vi "auto_rampnav.vi"(11 "Distance":dbl=7000.0) -> (3 "Complete":bool)   [LabVIEW 2010, in "LASA Beta.lvrbt"]
uses:
  LASA Beta.lvrbt
  op-run.vi
  op-read.vi
  <vilib>/NXT/Dual Mode Library/Display/drawNumber.vi
  <vilib>/NXT/Dual Mode Library/Display/drawText_center.vi
  <vilib>/NXT/Dual Mode Library/Waits/Wait_Num(msec).vi
panel:
  in  "Speed":dbl=40.0
  # "Measured in encoder counts, from wall start to 4th box"
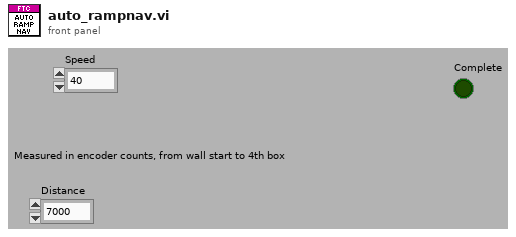
[diagram p1: front panel]
types:
  T1 = enum16{"Move Forward", "Move Left", "Allign To Ramp", "Orient To Ramp", "Climb Ramp", "Exit"}
  T2 = typedef "LVHSConnector.ctl" = cluster{"Hardware":string, "Flattened String":string}
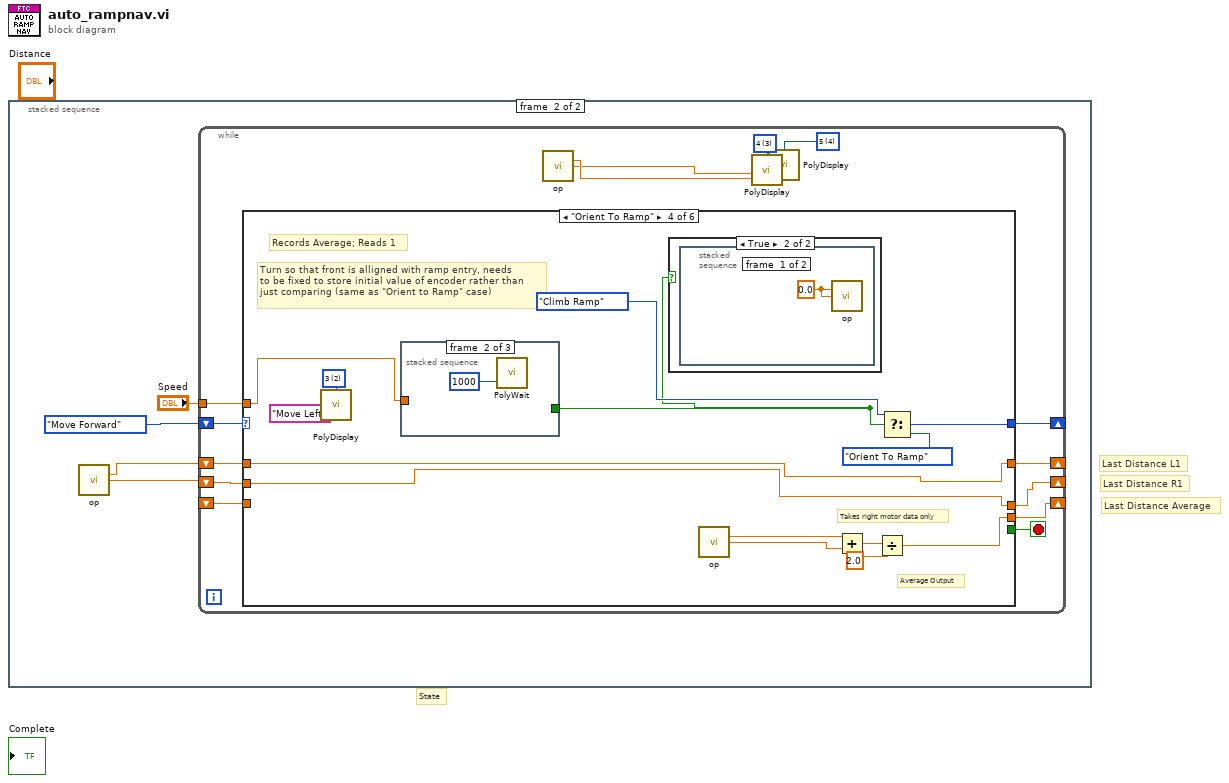
[diagram p0: block diagram]
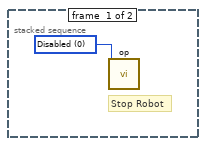
[diagram p2: hidden frame]
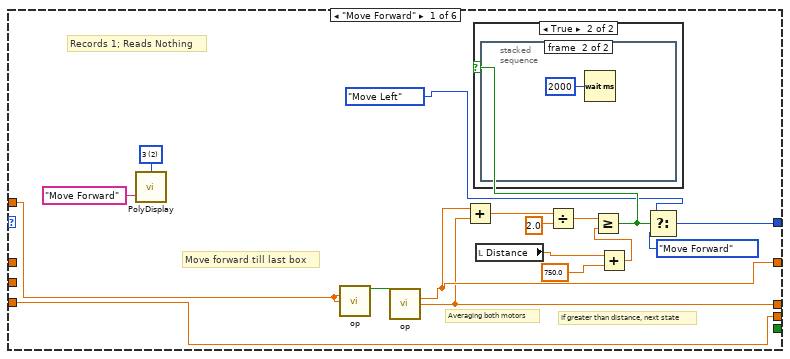
[diagram p3: hidden frame]
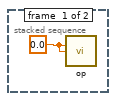
[diagram p5: hidden frame]
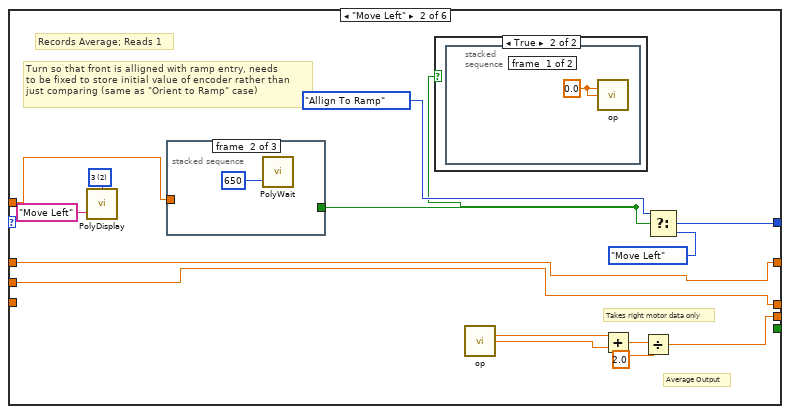
[diagram p6: hidden frame]
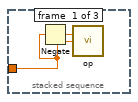
[diagram p7: hidden frame]
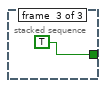
[diagram p8: hidden frame]
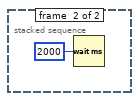
[diagram p10: hidden frame]
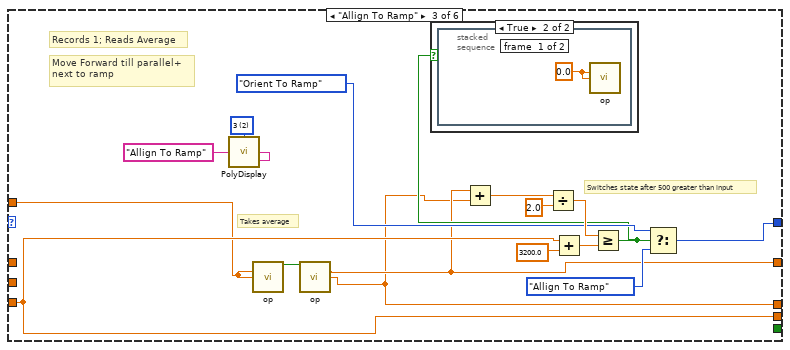
[diagram p11: hidden frame]
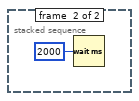
[diagram p13: hidden frame]
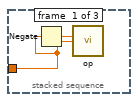
[diagram p14: hidden frame]
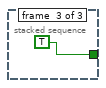
[diagram p15: hidden frame]
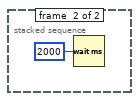
[diagram p17: hidden frame]
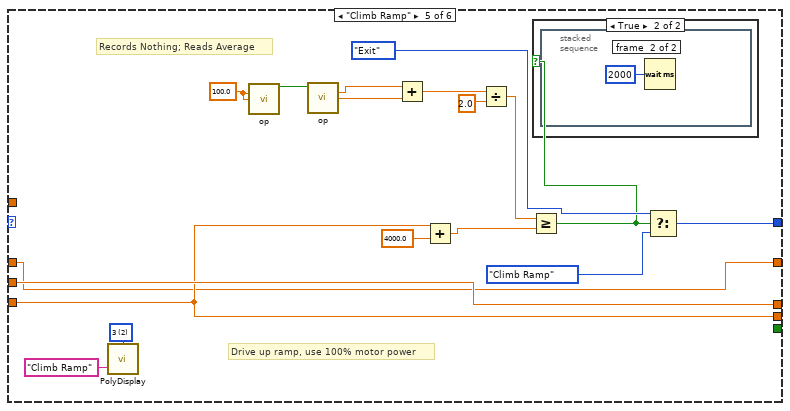
[diagram p18: hidden frame]
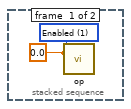
[diagram p20: hidden frame]
diagram:
  # "Last Distance Average"
  # "Last Distance R1"
  # "Last Distance L1"
  # "State"
  n1 = stacked-sequence {
    frame #0 {
      w1 = u16 0 items=["Disabled", "Enabled", "Initialize", "Read Only"] ("Status")
      # "Stop Robot"
      n2 = call-poly "op.vi"("Left Drive"=w1) -> ()  [unwired: 14 in, 1 out]
    }
    frame #1 {
      n3 = call-poly "op.vi"() -> ("Encoder Left Drive"=w4:dbl, "Encoder Right Drive"=w3:dbl)  [unwired: 9 in, 5 out]
      n4 = while {
        shift-right: [w19] -> _
        shift-left: T1."Move Forward" -> [w20]
        shift-right: [w8] -> _
        shift-left: w4 -> [w17]
        shift-right: [w12] -> _
        shift-left: w3 -> [w16]
        shift-right: [w11] -> _
        shift-left: _ -> [w15]
        tunnel: "Speed" -> [w6]
        stop <- w18 stop-if-true
        w13 = i16 4 items=["1", "2", "3", "4", "5", "6", "7", "8"] ("Line")
        w14 = i16 3 items=["1", "2", "3", "4", "5", "6", "7", "8"] ("Line")
        n5 = case shown="\"Orient To Ramp\"" w20 {
          tunnel: [w34 w52 w71 w90 w110 T1."Exit"] -> w19
          tunnel: [_ _ _ _ _ w125] -> w18
          tunnel: w17 -> [_ w42 _ w80 w98 w120]
          tunnel: [w23 w48 w61 w86 w107 w124] -> w12
          tunnel: [w32 w50 w68 w88 w106 w123] -> w11
          tunnel: w16 -> [_ w48 _ w86 w107 w124]
          tunnel: w15 -> [w32 _ w68 _ w106 w123]
          tunnel: [w24 w42 w62 w80 w98 w120] -> w8
          tunnel: w6 -> [w21 w40 w60 w78 _ _]
          frame "Move Forward" {
            w31 = i16 2 items=["1", "2", "3", "4", "5", "6", "7", "8"] ("Line")
            # "If greater than distance, next state"
            # "Averaging both motors"
            # "Records 1; Reads Nothing"
            # "Move forward till last box"
            n6 = call-poly <vilib>:"PolyDisplay.vi"("Text"="Move Forward", "Line"=w31) -> ()  [unwired: 2 in, 1 out]
            n7 = call-poly "op.vi"("Left Drive"=w21, "Right Drive"=w21) -> ("Chain OUT"=w22:bool)  [unwired: 13 in]
            n8 = call-poly "op.vi"("Chain IN"=w22) -> ("Encoder Left Drive"=w24:dbl, "Encoder Right Drive"=w23:dbl)  [unwired: 8 in, 5 out]
            n9 = Add(x=w24, y=w23) -> (x+y=w37:dbl)
            n10 = local read "Distance"() -> (w27:dbl)
            n11 = Divide(x=w37, y=2.0) -> (x/y=w33:dbl)
            n12 = Add(x=w27, y=750.0) -> (x+y=w25:dbl)
            n13 = Greater Or Equal?(x=w33, y=w25) -> (x >= y?=w29:bool)
            n14 = case shown="True" w29 {
              frame False {
              }
              frame True {
                n15 = stacked-sequence {
                  frame #0 {
                    w38 = 0.0 ("y")
                    n16 = call-poly "op.vi"("Left Drive"=w38, "Right Drive"=w38) -> ()  [unwired: 13 in, 1 out]
                  }
                  frame #1 {
                    n17 = Wait (ms)(milliseconds to wait=u32 2000) -> ()  [unwired: 1 out]
                  }
                }
              }
            }
            n18 = Select(t=T1."Move Left", s=w29, f=T1."Move Forward") -> (s? t:f=w34:T1)
          }
          frame "Move Left" {
            w47 = i16 2 items=["1", "2", "3", "4", "5", "6", "7", "8"] ("Line")
            # "Takes right motor data only"
            # "Average Output"
            # "Records Average; Reads 1"
            # "Turn so that front is alligned with ramp entry, needs\nto be fixed to store initial value of encoder rather than \njust comparing (same as \"Orient to Ramp\" case)"
            n19 = call-poly <vilib>:"PolyDisplay.vi"("Text"="Move Left", "Line"=w47) -> ()  [unwired: 2 in, 1 out]
            n20 = stacked-sequence {
              tunnel: [_ _ TRUE] -> w41
              tunnel: w40 -> [w55 _ _]
              frame #0 {
                n21 = Negate(x=w55) -> (-x=w54:dbl)
                n22 = call-poly "op.vi"("Left Drive"=w54, "Right Drive"=w55) -> ()  [unwired: 13 in, 1 out]
              }
              frame #1 {
                n23 = call-poly <vilib>:"PolyWait.vi"("Time (100 msec)"=u32 650) -> ()  [unwired: 3 in, 1 out]
              }
              frame #2 {
              }
            }
            n24 = case shown="True" w41 {
              frame False {
              }
              frame True {
                n25 = stacked-sequence {
                  frame #0 {
                    w58 = 0.0 ("y")
                    n26 = call-poly "op.vi"("Left Drive"=w58, "Right Drive"=w58) -> ()  [unwired: 13 in, 1 out]
                  }
                  frame #1 {
                    n27 = Wait (ms)(milliseconds to wait=u32 2000) -> ()  [unwired: 1 out]
                  }
                }
              }
            }
            n28 = call-poly "op.vi"() -> ("Encoder Left Drive"=w44:dbl, "Encoder Right Drive"=w43:dbl)  [unwired: 9 in, 5 out]
            n29 = Add(x=w44, y=w43) -> (x+y=w51:dbl)
            n30 = Divide(x=w51, y=2.0) -> (x/y=w50:dbl)
            n31 = Select(t=T1."Allign To Ramp", s=w41, f=T1."Move Left") -> (s? t:f=w52:T1)
          }
          frame "Allign To Ramp" {
            w67 = i16 2 items=["1", "2", "3", "4", "5", "6", "7", "8"] ("Line")
            # "Switches state after 500 greater than input"
            # "Takes average"
            # "Records 1; Reads Average"
            # "Move Forward till parallel+\nnext to ramp"
            n32 = call-poly <vilib>:"PolyDisplay.vi"("Text"="Allign To Ramp", "Line"=w67) -> ()  [unwired: 2 in, 1 out]
            n33 = call-poly "op.vi"("Left Drive"=w60, "Right Drive"=w60) -> ("Chain OUT"=w63:bool)  [unwired: 13 in]
            n34 = call-poly "op.vi"("Chain IN"=w63) -> ("Encoder Left Drive"=w62:dbl, "Encoder Right Drive"=w61:dbl)  [unwired: 8 in, 5 out]
            n35 = Add(x=w62, y=w61) -> (x+y=w75:dbl)
            n36 = Divide(x=w75, y=2.0) -> (x/y=w73:dbl)
            n37 = Add(x=w68, y=3200.0) -> (x+y=w70:dbl)
            n38 = Greater Or Equal?(x=w73, y=w70) -> (x >= y?=w64:bool)
            n39 = case shown="True" w64 {
              frame False {
              }
              frame True {
                n40 = stacked-sequence {
                  frame #0 {
                    w76 = 0.0 ("y")
                    n41 = call-poly "op.vi"("Left Drive"=w76, "Right Drive"=w76) -> ()  [unwired: 13 in, 1 out]
                  }
                  frame #1 {
                    n42 = Wait (ms)(milliseconds to wait=u32 2000) -> ()  [unwired: 1 out]
                  }
                }
              }
            }
            n43 = Select(t=T1."Orient To Ramp", s=w64, f=T1."Allign To Ramp") -> (s? t:f=w71:T1)
          }
          frame "Orient To Ramp" {
            w85 = i16 2 items=["1", "2", "3", "4", "5", "6", "7", "8"] ("Line")
            # "Takes right motor data only"
            # "Average Output"
            # "Records Average; Reads 1"
            # "Turn so that front is alligned with ramp entry, needs\nto be fixed to store initial value of encoder rather than \njust comparing (same as \"Orient to Ramp\" case)"
            n44 = call-poly <vilib>:"PolyDisplay.vi"("Text"="Move Left", "Line"=w85) -> ()  [unwired: 2 in, 1 out]
            n45 = stacked-sequence {
              tunnel: [_ _ TRUE] -> w79
              tunnel: w78 -> [w93 _ _]
              frame #0 {
                n46 = Negate(x=w93) -> (-x=w92:dbl)
                n47 = call-poly "op.vi"("Left Drive"=w92, "Right Drive"=w93) -> ()  [unwired: 13 in, 1 out]
              }
              frame #1 {
                n48 = call-poly <vilib>:"PolyWait.vi"("Time (100 msec)"=u32 1000) -> ()  [unwired: 3 in, 1 out]
              }
              frame #2 {
              }
            }
            n49 = case shown="True" w79 {
              frame False {
              }
              frame True {
                n50 = stacked-sequence {
                  frame #0 {
                    w96 = 0.0 ("y")
                    n51 = call-poly "op.vi"("Left Drive"=w96, "Right Drive"=w96) -> ()  [unwired: 13 in, 1 out]
                  }
                  frame #1 {
                    n52 = Wait (ms)(milliseconds to wait=u32 2000) -> ()  [unwired: 1 out]
                  }
                }
              }
            }
            n53 = call-poly "op.vi"() -> ("Encoder Left Drive"=w82:dbl, "Encoder Right Drive"=w81:dbl)  [unwired: 9 in, 5 out]
            n54 = Add(x=w82, y=w81) -> (x+y=w89:dbl)
            n55 = Divide(x=w89, y=2.0) -> (x/y=w88:dbl)
            n56 = Select(t=T1."Climb Ramp", s=w79, f=T1."Orient To Ramp") -> (s? t:f=w90:T1)
          }
          frame "Climb Ramp" {
            w105 = i16 2 items=["1", "2", "3", "4", "5", "6", "7", "8"] ("Line")
            w112 = 100.0 ("Left Drive")
            # "Records Nothing; Reads Average"
            # "Drive up ramp, use 100% motor power"
            n57 = call-poly <vilib>:"PolyDisplay.vi"("Text"="Climb Ramp", "Line"=w105) -> ()  [unwired: 2 in, 1 out]
            n58 = call-poly "op.vi"("Left Drive"=w112, "Right Drive"=w112) -> ("Chain OUT"=w101:bool)  [unwired: 13 in]
            n59 = call-poly "op.vi"("Chain IN"=w101) -> ("Encoder Left Drive"=w100:dbl, "Encoder Right Drive"=w99:dbl)  [unwired: 8 in, 5 out]
            n60 = Add(x=w100, y=w99) -> (x+y=w115:dbl)
            n61 = Add(x=w106, y=4000.0) -> (x+y=w108:dbl)
            n62 = Divide(x=w115, y=2.0) -> (x/y=w113:dbl)
            n63 = Greater Or Equal?(x=w113, y=w108) -> (x >= y?=w102:bool)
            n64 = case shown="True" w102 {
              frame False {
              }
              frame True {
                n65 = stacked-sequence {
                  frame #0 {
                    w116 = 0.0 ("y")
                    w117 = u16 1 items=["Disabled", "Enabled", "Initialize", "Read Only"] ("Status")
                    n66 = call-poly "op.vi"("Left Drive"=w116, "Right Drive"=w116, "Arm"=w117) -> ()  [unwired: 12 in, 1 out]
                  }
                  frame #1 {
                    n67 = Wait (ms)(milliseconds to wait=u32 2000) -> ()  [unwired: 1 out]
                  }
                }
              }
            }
            n68 = Select(t=T1."Exit", s=w102, f=T1."Climb Ramp") -> (s? t:f=w110:T1)
          }
          frame "Exit", Default {
            w119 = 0.0 ("Left Drive")
            w122 = i16 2 items=["1", "2", "3", "4", "5", "6", "7", "8"] ("Line")
            w125 = TRUE
            n69 = call-poly <vilib>:"PolyDisplay.vi"("Text"="Exit", "Line"=w122) -> ()  [unwired: 2 in, 1 out]
            n70 = call-poly "op.vi"("Left Drive"=w119, "Right Drive"=w119) -> ()  [unwired: 13 in, 1 out]
            n71 = local write "Complete"(w125) -> ()
          }
        }
        n72 = call-poly "op.vi"() -> ("Encoder Left Drive"=w10:dbl, "Encoder Right Drive"=w9:dbl)  [unwired: 9 in, 5 out]
        n73 = call-poly <vilib>:"PolyDisplay.vi"("number"=w10, "Line"=w14) -> ("NXT"=w7:T2)  [unwired: 2 in]
        n74 = call-poly <vilib>:"PolyDisplay.vi"("number"=w9, "NXT"=w7, "Line"=w13) -> ()  [unwired: 1 in, 1 out]
      }
    }
  }
